vi "Create waveform.vi"(4 "Seconds to read":dbl, 6 "Complete File?":bool, 7 "Reading Interface":enum32{"Read MP3", "Read generated waveform"}(tab), 8 "error in":errorcluster, 9 "Generated Signal Configuration":T1={"signal type"=enum."Sine Wave", "frequency"=1000.0, "sampling info"={"Sampling Rate"=44100.0, "# Samples"=10000.0}} {"frequency" format="%#_13g"}, 10 "Input File":path) -> (0 "error out":errorcluster, 2 "output waveform":waveform(dbl))   [LabVIEW 2014, in "Melody Extraction.lvlib"]
uses:
  Melody Extraction.lvlib
  <vilib>/measure/NI_MABase.lvlib
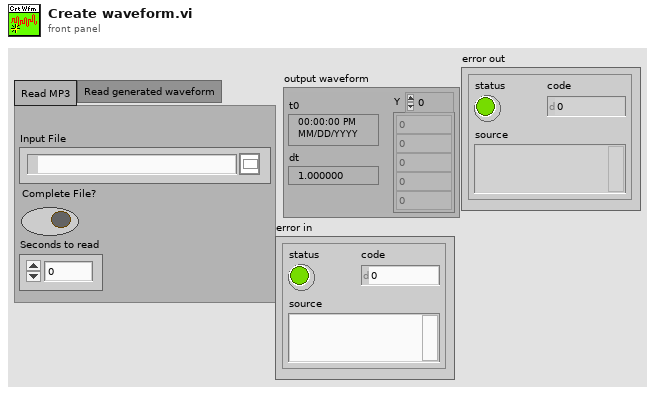
[diagram p1: front panel]
types:
  T1 = cluster{"signal type":enum16{"Sine Wave", "Triangle Wave", "Square Wave", "Sawtooth Wave"}, "frequency":dbl, "sampling info":cluster{"Sampling Rate":dbl, "# Samples":dbl}}
  T2 = enum16{"Sine Wave", "Triangle Wave", "Square Wave", "Sawtooth Wave"}
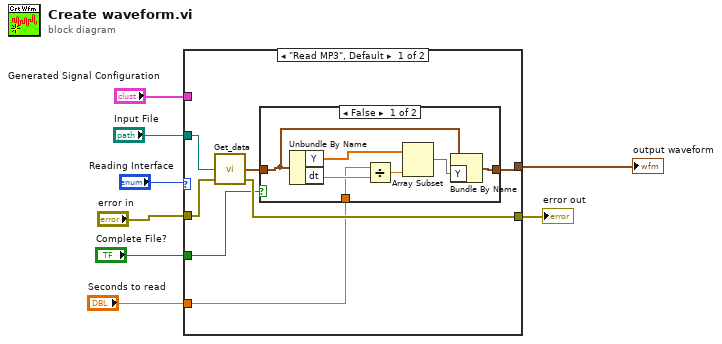
[diagram p0: block diagram]
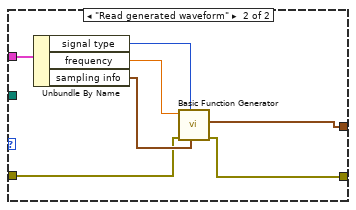
[diagram p3: hidden frame]
diagram:
  n1 = case shown="\"Read MP3\", Default" "Reading Interface" {
    tunnel: "Input File" -> [w15 _]
    tunnel: "Generated Signal Configuration" -> [_ w30]
    tunnel: "error in" -> [w14 w26]
    tunnel: [w13 w25] -> w5
    tunnel: [w10 w24] -> w3
    tunnel: "Complete File?" -> [w12 _]
    tunnel: "Seconds to read" -> [w9 _]
    frame "Read MP3", Default {
      n2 = call "Get_data.vi"("error in (no error)"=w14, "Input File"=w15) -> ("error out"=w13:errorcluster, "Output Waveform"=w11:waveform(dbl))  [unwired: 2 in]
      n3 = case shown="False" w12 {
        tunnel: w11 -> [w17 w23]
        tunnel: [w16 w23] -> w10
        tunnel: w9 -> [w21 _]
        frame False {
          n4 = Unbundle By Name(w17) -> ("Y"=w19:dbl[], "dt"=w22:dbl)
          n5 = Divide(x=w21, y=w22) -> (x/y=w20:dbl)
          n6 = Array Subset(array=w19, length=w20) -> (w18:dbl[])  [unwired: 1 in]
          n7 = Bundle By Name(cluster=w17, "Y"=w18) -> (w16:waveform(dbl))
        }
        frame True {
        }
      }
    }
    frame "Read generated waveform" {
      n8 = Unbundle By Name(w30) -> ("signal type"=w29:T2, "frequency"=w28:dbl, "sampling info"=w27:cluster{"Sampling Rate":dbl, "# Samples":dbl})
      n9 = call <vilib>:"Basic Function Generator.vi"("sampling info"=w27, "signal type"=w29, "error in (no error)"=w26, "frequency"=w28) -> ("error out"=w25:errorcluster, "signal out"=w24:waveform(dbl))  [unwired: 5 in, 1 out]
    }
  }
  "output waveform" <- w3
  "error out" <- w5
